vi "EnablePTO.vi"(8 "error in (no error)":errorcluster) -> (0 "error out":errorcluster)   [LabVIEW 2015]
uses:
  Solenoids/Solenoids.ctl
  <vilib>/Rock Robotics/WPI/Solenoid/WPI_SolenoidValue.ctl
  Framework/Robot Global Data.vi
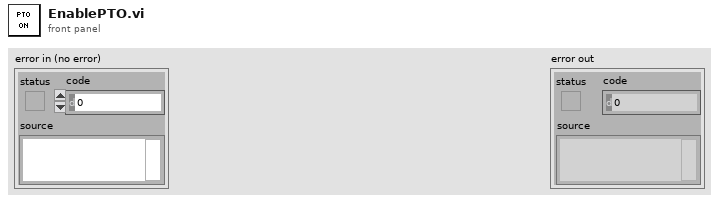
[diagram p1: front panel]
types:
  T1 = typedef "WPI_SolenoidValue.ctl" = enum16{"Off", "On", "Forward", "Reverse"}
  T2 = typedef "Solenoids.ctl" = enum16{"Gear Low", "Gear High", "Shoot Ball", "Hold Ball", "PTO Active", "PTO De-Active"}
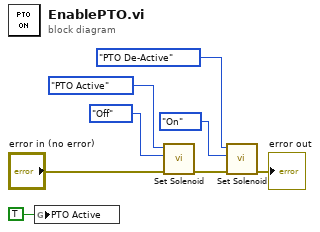
[diagram p0: block diagram]
diagram:
  n1 = global write "Robot Global Data.vi" "PTO Active"(TRUE) -> ()
  n2 = call "Set Solenoid.vi"("error in (no error)"="error in (no error)", "Value"=WPI_SolenoidValue."Off", "Solenoids"=Solenoids."PTO Active") -> ("error out"=w3:errorcluster)  [unwired: 8 in]
  n3 = call "Set Solenoid.vi"("error in (no error)"=w3, "Value"=WPI_SolenoidValue."On", "Solenoids"=Solenoids."PTO De-Active") -> ("error out"=→"error out":errorcluster)  [unwired: 8 in]
